vi "Suck ball.vi"(2 "error in (no error)":errorcluster) -> (0 "error out":errorcluster)   [LabVIEW 2013]
uses:
  InTake Global Data.vi
  Cannon/Cannon Global Data.vi
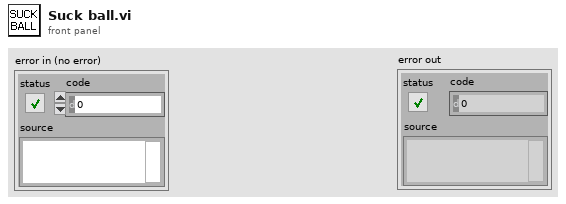
[diagram p1: front panel]
types:
  T1 = cluster{"TakeBall":dbl, "UpperClaw":dbl, "LowerClaw":dbl, "MS":bool, "Upper claw max":bool, "Lower claw max":bool, "Upper claw min":bool, "Lower claw min":bool, "Angle":dbl}
  T2 = typedef "WPI_SolenoidValue.ctl" = enum16{"Off", "On", "Forward", "Reverse"}
  T3 = cluster{"MS":bool, "Shoot!":T2, "Angle":dbl, "Reset Gyro?":bool}
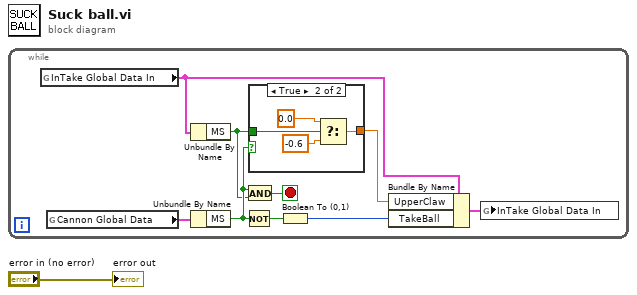
[diagram p0: block diagram]
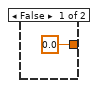
[diagram p2: hidden frame]
diagram:
  n1 = while {
    stop <- w2 stop-if-true
    n2 = global read "InTake Global Data.vi" "InTake Global Data In"() -> (w10:T1)
    n3 = global read "Cannon Global Data.vi" "Cannon Global Data"() -> (w7:T3)
    n4 = Unbundle By Name(w10) -> ("MS"=w3:bool)
    n5 = Unbundle By Name(w7) -> ("MS"=w4:bool)
    n6 = Not(x=w4) -> (.not. x?=w9:bool)
    n7 = And(x=w4, y=w3) -> (x .and. y?=w2:bool)
    n8 = case shown="True" w4 {
      tunnel: [0.0 w15] -> w5
      tunnel: w3 -> [_ w14]
      frame False {
      }
      frame True {
        n9 = Select(t=0.0 ("f"), s=w14, f=-0.6) -> (s? t:f=w15:dbl)
      }
    }
    n10 = Boolean To (0,1)(Boolean=w9) -> (0, 1=w6:i16)
    n11 = Bundle By Name(cluster=w10, "UpperClaw"=w5, "TakeBall"=w6) -> (w8:T1)
    n12 = global write "InTake Global Data.vi" "InTake Global Data In"(w8) -> ()
  }
  "error out" <- "error in (no error)"
